vi "Elevator.vi"() -> ()   [LabVIEW 2019]
uses:
  <vilib>/Rock Robotics/WPI/ThirdParty/Phoenix-LabVIEW/Motor Controller/Controls/CTRE_Phoenix_MotorControl_ControlMode.ctl
  <vilib>/Rock Robotics/WPI/Utilities/WPI_GetSetVariantRefNum.vi
  <vilib>/Rock Robotics/Network Tables/NT Write Boolean.vi
panel:
  out "climb":bool
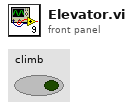
[diagram p1: front panel]
types:
  T1 = typedef "WPI_JoystickDevRef.ctl" = cluster{"Device":T2}
  T2 = typedef "WPI_JoystickDeviceEnum.ctl" = enum16{"USB 0", "USB 1", "USB 2", "USB 3", "USB 4", "USB 5"}
  T3 = typedef "WPI_MotorControlDeviceRef.ctl" = cluster{"DeviceStatus":errorcluster, "Type":T4, "PWM":cluster{"PWM Channel":T5, "DeadBand":T6}, "CAN":cluster{"Device Number":u8, "SetOutput VI Ref":variant, "GetOutput VI Ref":variant, "Enable VI Ref":variant, "Disable VI Ref":variant, "Data":variant}, "Invert":bool, "DIO PWM":cluster{"PWM \"Enable\" Channel":T5, "DIOChannel":T7, "PWM Rate":dbl}}
  T4 = typedef "WPI_MotorControlType.ctl" = enum16{"PWM", "CAN", "DIO PWM"}
  T5 = typedef "FPGA_DIOPWMChannel.ctl" = enum8{"PWM 0", "PWM 1", "PWM 2", "PWM 3", "PWM 4", "PWM 5", "PWM 6", "PWM 7", "PWM 8", "PWM 9", "PWM MXP 0", "PWM MXP 1", "PWM MXP 2", "PWM MXP 3", "PWM MXP 4", "PWM MXP 5", "PWM MXP 6", "PWM MXP 7", "PWM MXP 8", "PWM MXP 9", "Invalid"}
  T6 = typedef "WPI_PWMDeadband.ctl" = cluster{"Name":string, "maxPositivePwm":i32, "minPositivePwm":i32, "centerPwm":i32, "maxNegativePwm":i32, "minNegativePwm":i32, "angularRange":u16}
  T7 = typedef "FPGA_DIOChannel.ctl" = enum8{"DIO 0", "DIO 1", "DIO 2", "DIO 3", "DIO 4", "DIO 5", "DIO 6", "DIO 7", "DIO 8", "DIO 9", "DIO MXP 0", "DIO MXP 1", "DIO MXP 2", "DIO MXP 3", "DIO MXP 4", "DIO MXP 5", "DIO MXP 6", "DIO MXP 7", "DIO MXP 8", "DIO MXP 9", "DIO MXP 10", "DIO MXP 11", "DIO MXP 12", "DIO MXP 13", "DIO MXP 14", "DIO MXP 15", "SPI Port CS1", "SPI Port CS2", "SPI Port CS3", "SPI Port MISO", "SPI Port MOSI", "Invalid"}
  T8 = typedef "CTRE_Phoenix_MotorControl_ControlMode.ctl" = u16
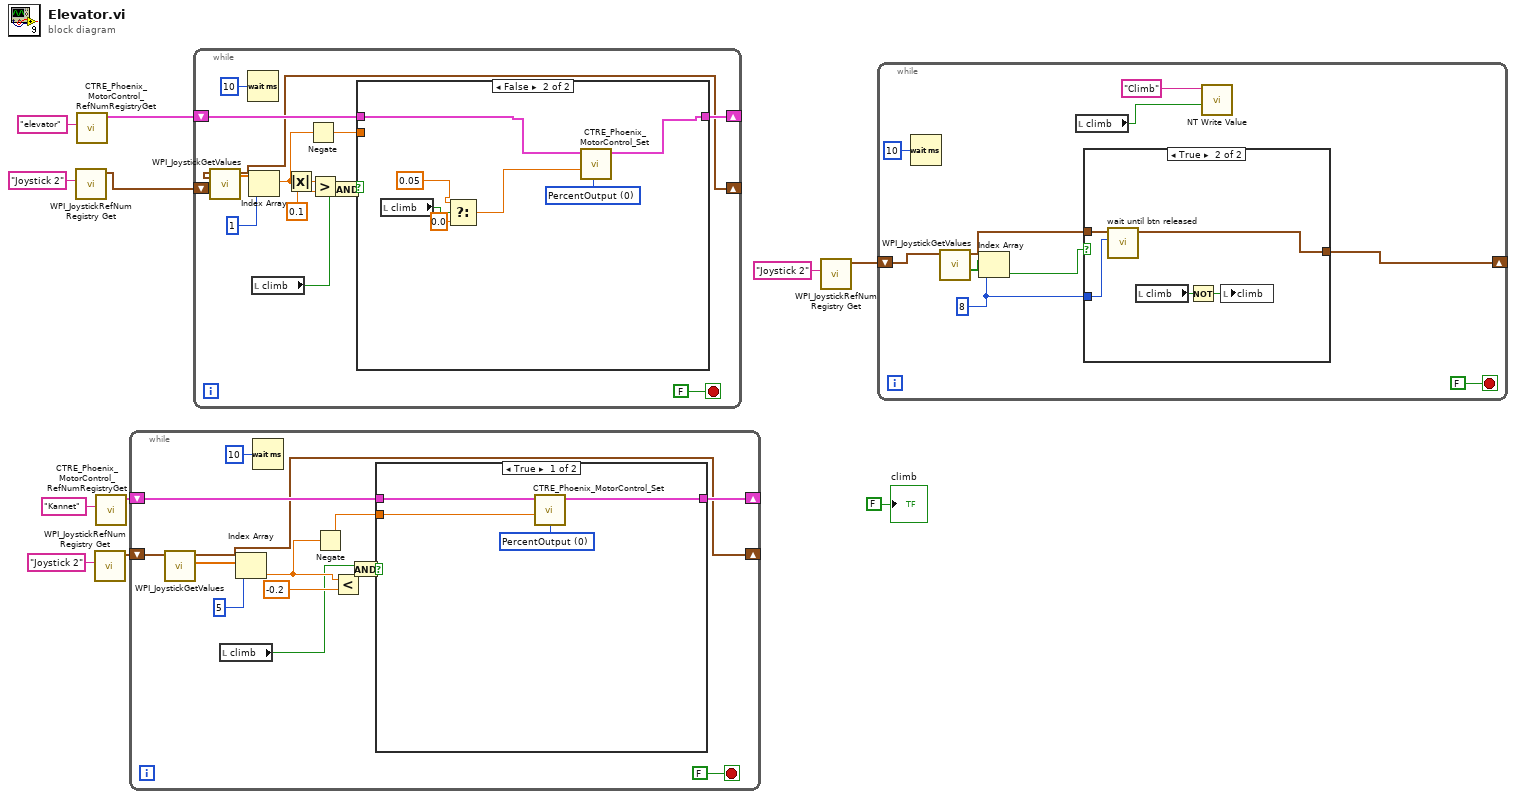
[diagram p0: block diagram]
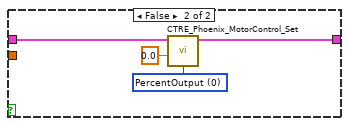
[diagram p3: hidden frame]
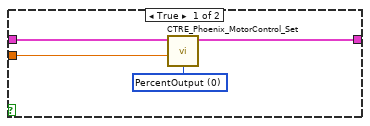
[diagram p4: hidden frame]
diagram:
  n1 = call <vilib>:"WPI_JoystickRefNum Registry Get.vi"("refnum name"="Joystick 2") -> ("JoystickDevRef"=w11:T1)  [unwired: 9 in, 1 out]
  n2 = call <vilib>:"CTRE_Phoenix_MotorControl_RefNumRegistryGet.vi"("refnum name"="elevator") -> ("PhoenixMotorControlDevRef"=w9:T3)  [unwired: 9 in, 1 out]
  n3 = call <vilib>:"WPI_JoystickRefNum Registry Get.vi"("refnum name"="Joystick 2") -> ("JoystickDevRef"=w7:T1)  [unwired: 9 in, 1 out]
  n4 = call <vilib>:"CTRE_Phoenix_MotorControl_RefNumRegistryGet.vi"("refnum name"="Kannet") -> ("PhoenixMotorControlDevRef"=w5:T3)  [unwired: 9 in, 1 out]
  n5 = while {
    shift-right: [w23] -> _
    shift-left: w5 -> [w22]
    shift-right: [w19] -> _
    shift-left: w7 -> [w25]
    stop <- FALSE stop-if-true
    n6 = call <vilib>:"WPI_JoystickGetValues.vi"("JoystickDevRef"=w25) -> ("Axes"=w18:dbl[], "JoystickDevRef"=w19:T1)  [unwired: 6 in, 3 out]
    n7 = local read "climb"() -> (w12:bool)
    n8 = Index Array(array=w18, index=5) -> (element=w15:dbl)
    n9 = Wait (ms)(milliseconds to wait=u32 10) -> ()  [unwired: 1 out]
    n10 = Negate(x=w15) -> (-x=w14:dbl)
    n11 = Less?(x=w15, y=-0.2) -> (x < y?=w17:bool)
    n12 = And(x=w12, y=w17) -> (x .and. y?=w13:bool)
    n13 = case shown="True" w13 {
      tunnel: [w28 w32] -> w23
      tunnel: w22 -> [w29 w33]
      tunnel: w14 -> [w26 _]
      frame True {
        w27 = T8 0 items=["PercentOutput"=0, "Position"=1, "Velocity"=2, "Current"=3, "Follower"=5, "MotionProfile"=6, "MotionMagic"=7, "MotionProfileArc"=10, "Disabled"=15] ("Control Mode")
        n14 = call <vilib>:"CTRE_Phoenix_MotorControl_Set.vi"("Output"=w26, "Control Mode"=w27, "PhoenixMotorControlDevRef"=w29) -> ("PhoenixMotorControlDevRef"=w28:T3)  [unwired: 7 in, 1 out]
      }
      frame False {
        w31 = T8 0 items=["PercentOutput"=0, "Position"=1, "Velocity"=2, "Current"=3, "Follower"=5, "MotionProfile"=6, "MotionMagic"=7, "MotionProfileArc"=10, "Disabled"=15] ("Control Mode")
        n15 = call <vilib>:"CTRE_Phoenix_MotorControl_Set.vi"("Output"=0.0, "Control Mode"=w31, "PhoenixMotorControlDevRef"=w33) -> ("PhoenixMotorControlDevRef"=w32:T3)  [unwired: 7 in, 1 out]
      }
    }
  }
  n16 = while {
    shift-right: [w45] -> _
    shift-left: w9 -> [w44]
    shift-right: [w39] -> _
    shift-left: w11 -> [w48]
    stop <- FALSE stop-if-true
    n17 = call <vilib>:"WPI_JoystickGetValues.vi"("JoystickDevRef"=w48) -> ("Axes"=w47:dbl[], "JoystickDevRef"=w39:T1)  [unwired: 6 in, 3 out]
    n18 = Wait (ms)(milliseconds to wait=u32 10) -> ()  [unwired: 1 out]
    n19 = Index Array(array=w47, index=1) -> (element=w37:dbl)
    n20 = local read "climb"() -> (w34:bool)
    n21 = Absolute Value(x=w37) -> (abs(x)=w38:dbl)
    n22 = Negate(x=w37) -> (-x=w36:dbl)
    n23 = Greater?(x=w38, y=0.1) -> (0:w43:bool)
    n24 = And(x=w43, y=w34) -> (x .and. y?=w35:bool)
    n25 = case shown="False" w35 {
      tunnel: [w51 w58] -> w45
      tunnel: w44 -> [w52 w59]
      tunnel: w36 -> [w49 _]
      frame True {
        w50 = T8 0 items=["PercentOutput"=0, "Position"=1, "Velocity"=2, "Current"=3, "Follower"=5, "MotionProfile"=6, "MotionMagic"=7, "MotionProfileArc"=10, "Disabled"=15] ("Control Mode")
        n26 = call <vilib>:"CTRE_Phoenix_MotorControl_Set.vi"("Output"=w49, "Control Mode"=w50, "PhoenixMotorControlDevRef"=w52) -> ("PhoenixMotorControlDevRef"=w51:T3)  [unwired: 7 in, 1 out]
      }
      frame False {
        w57 = T8 0 items=["PercentOutput"=0, "Position"=1, "Velocity"=2, "Current"=3, "Follower"=5, "MotionProfile"=6, "MotionMagic"=7, "MotionProfileArc"=10, "Disabled"=15] ("Control Mode")
        n27 = local read "climb"() -> (w56:bool)
        n28 = Select(t=0.05 ("Output"), s=w56, f=0.0) -> (s? t:f=w53:dbl)
        n29 = call <vilib>:"CTRE_Phoenix_MotorControl_Set.vi"("Output"=w53, "Control Mode"=w57, "PhoenixMotorControlDevRef"=w59) -> ("PhoenixMotorControlDevRef"=w58:T3)  [unwired: 7 in, 1 out]
      }
    }
  }
  n30 = call <vilib>:"WPI_JoystickRefNum Registry Get.vi"("refnum name"="Joystick 2") -> ("JoystickDevRef"=w2:T1)  [unwired: 9 in, 1 out]
  n31 = while {
    shift-right: [w64] -> _
    shift-left: w2 -> [w67]
    stop <- FALSE stop-if-true
    w62 = 8 ("index")
    n32 = Wait (ms)(milliseconds to wait=u32 10) -> ()  [unwired: 1 out]
    n33 = call <vilib>:"WPI_JoystickGetValues.vi"("JoystickDevRef"=w67) -> ("Buttons"=w68:bool[], "JoystickDevRef"=w63:T1)  [unwired: 6 in, 3 out]
    n34 = Index Array(array=w68, index=w62) -> (element=w66:bool)
    n35 = local read "climb"() -> (w61:bool)
    n36 = case shown="True" w66 {
      tunnel: [w70 w72] -> w64
      tunnel: w63 -> [w70 w73]
      tunnel: w62 -> [_ w71]
      frame False {
      }
      frame True {
        n37 = call "wait until btn released.vi"("index"=w71, "JoystickDevRef"=w73) -> ("JoystickDevRef 2"=w72:T1)  [unwired: 9 in]
        n38 = local read "climb"() -> (w75:bool)
        n39 = Not(x=w75) -> (.not. x?=w74:bool)
        n40 = local write "climb"(w74) -> ()
      }
    }
    n41 = call-poly <vilib>:"NT Write Value.vi"("Boolean"=w61, "Name"="Climb") -> ()  [unwired: 9 in, 1 out]
  }
  "climb" <- FALSE ("climb")
